vi "TxData_Organization_EVM_Max.vi"() -> ()   [LabVIEW 2023, in "ParsingData.lvlib"]
uses:
  <vilib>/Utility/file.llb/Read Delimited Spreadsheet (string).vi
  <vilib>/Utility/file.llb/Read Delimited Spreadsheet (DBL).vi
  ParsingData.lvlib
panel:
  in  "File Path":path
  out "Max EVM : Mode       Polarity                     UD att                   BFIC COM               BFIC ele                  SG Power                EIRP                           EVM":string[](array[string])
  in  "Input power_up":dbl
  in  "Input power_low":dbl
  out "EVM to EIRP":cluster{dbl[], "all rows":dbl[]}[](graph)
  out "all rows":dbl[][](array[numeric])
  out "filenames":string[](array[string])
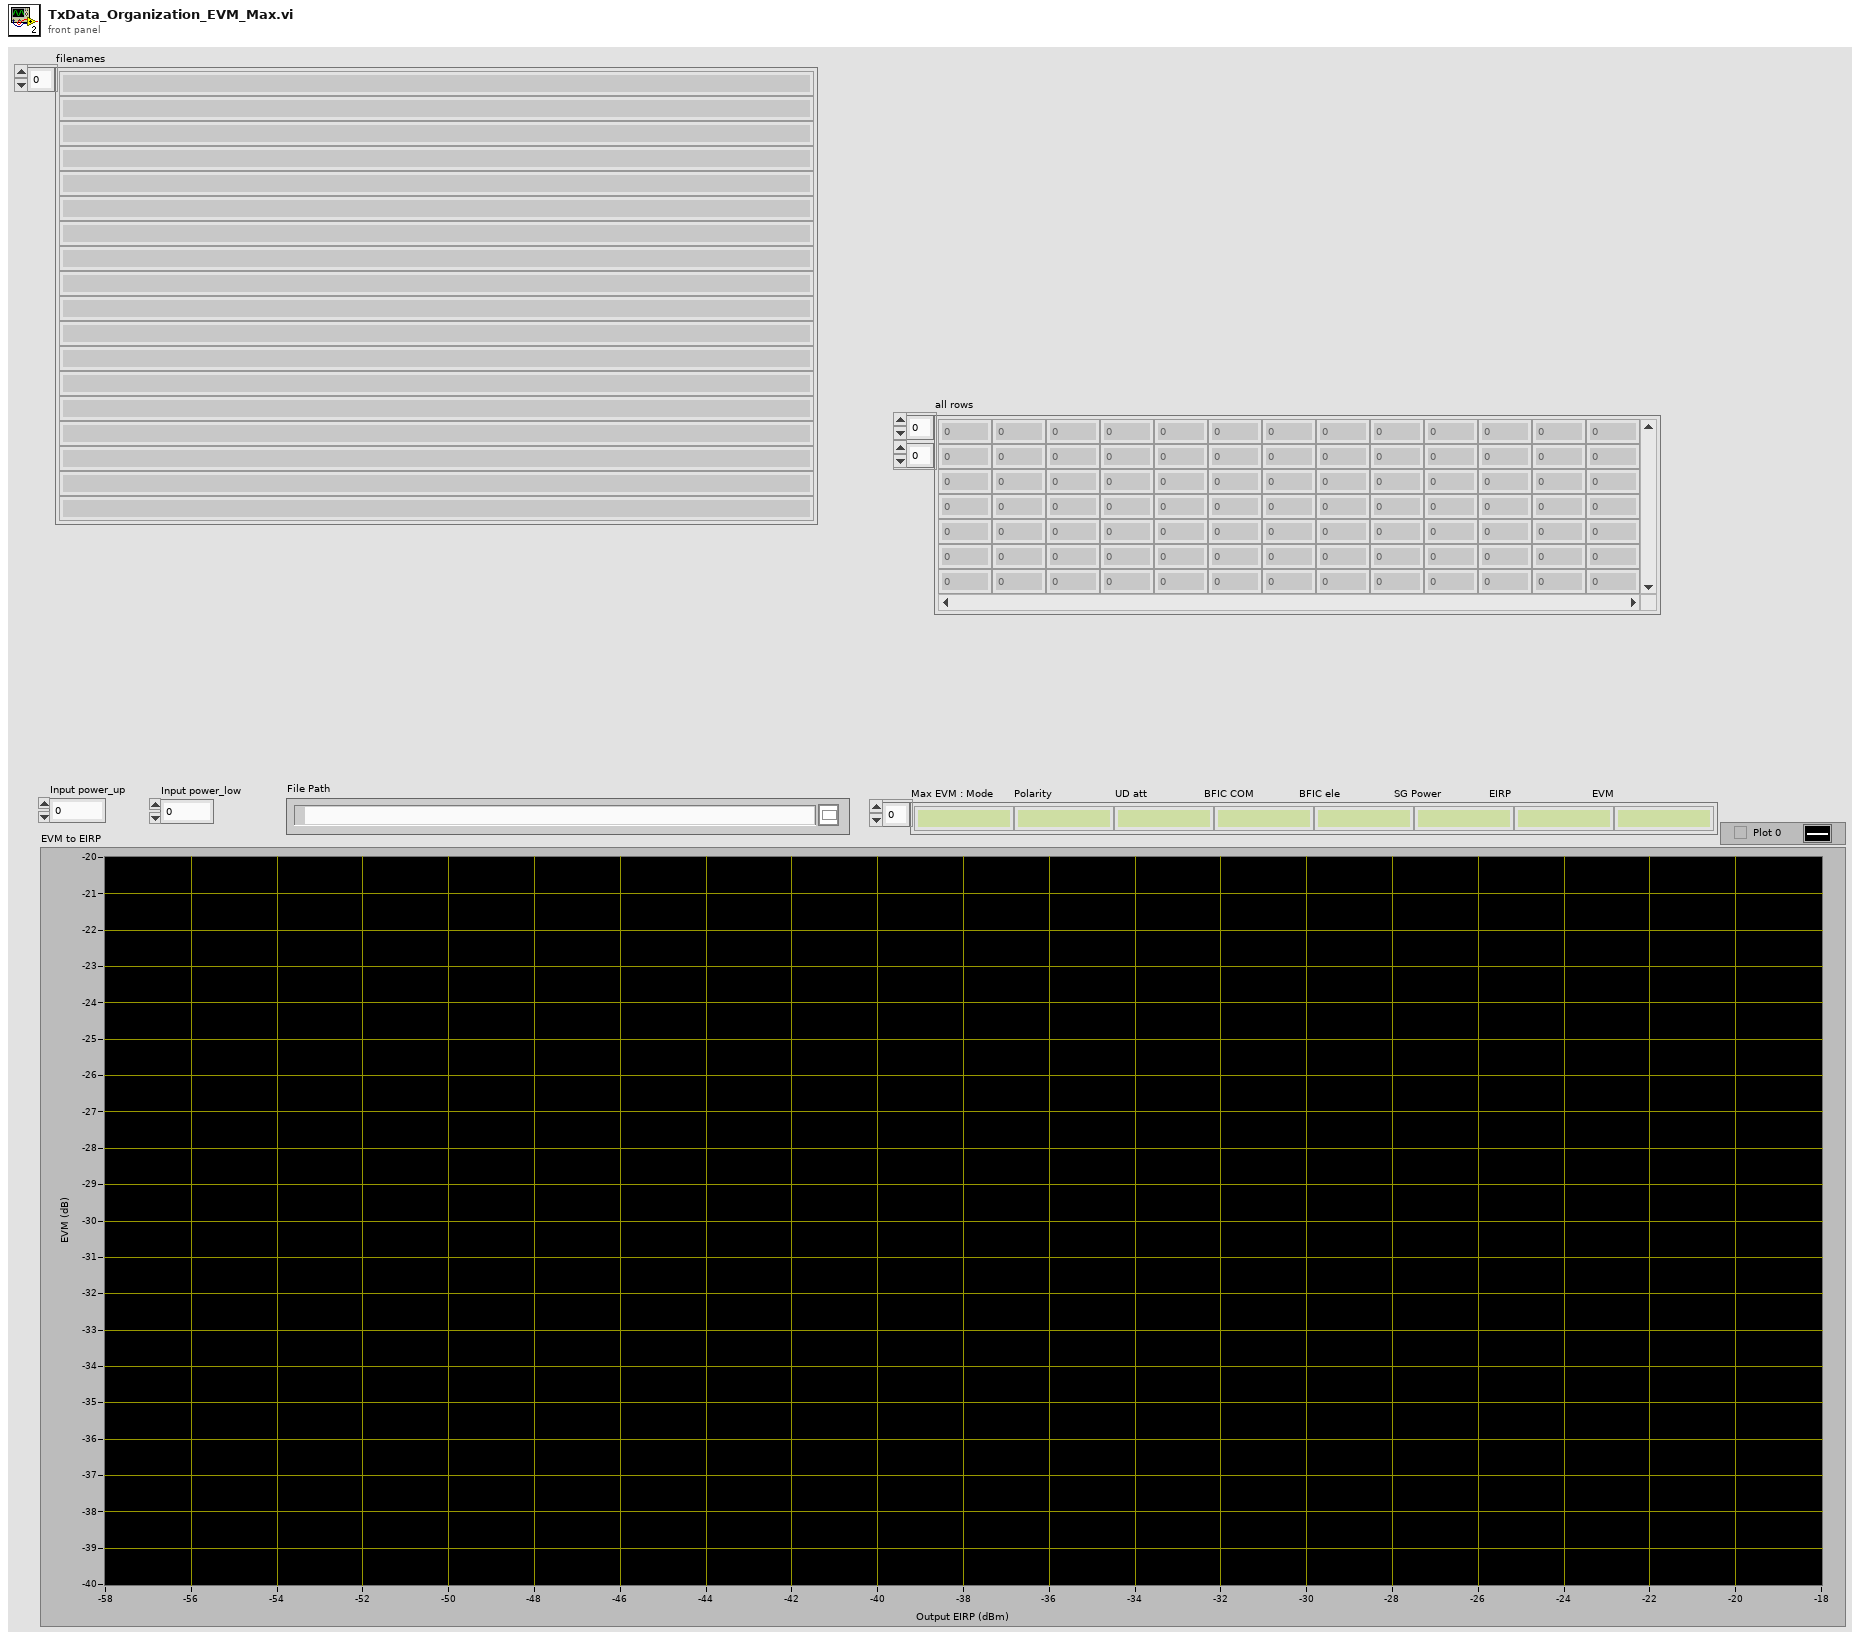
[diagram p1: front panel]
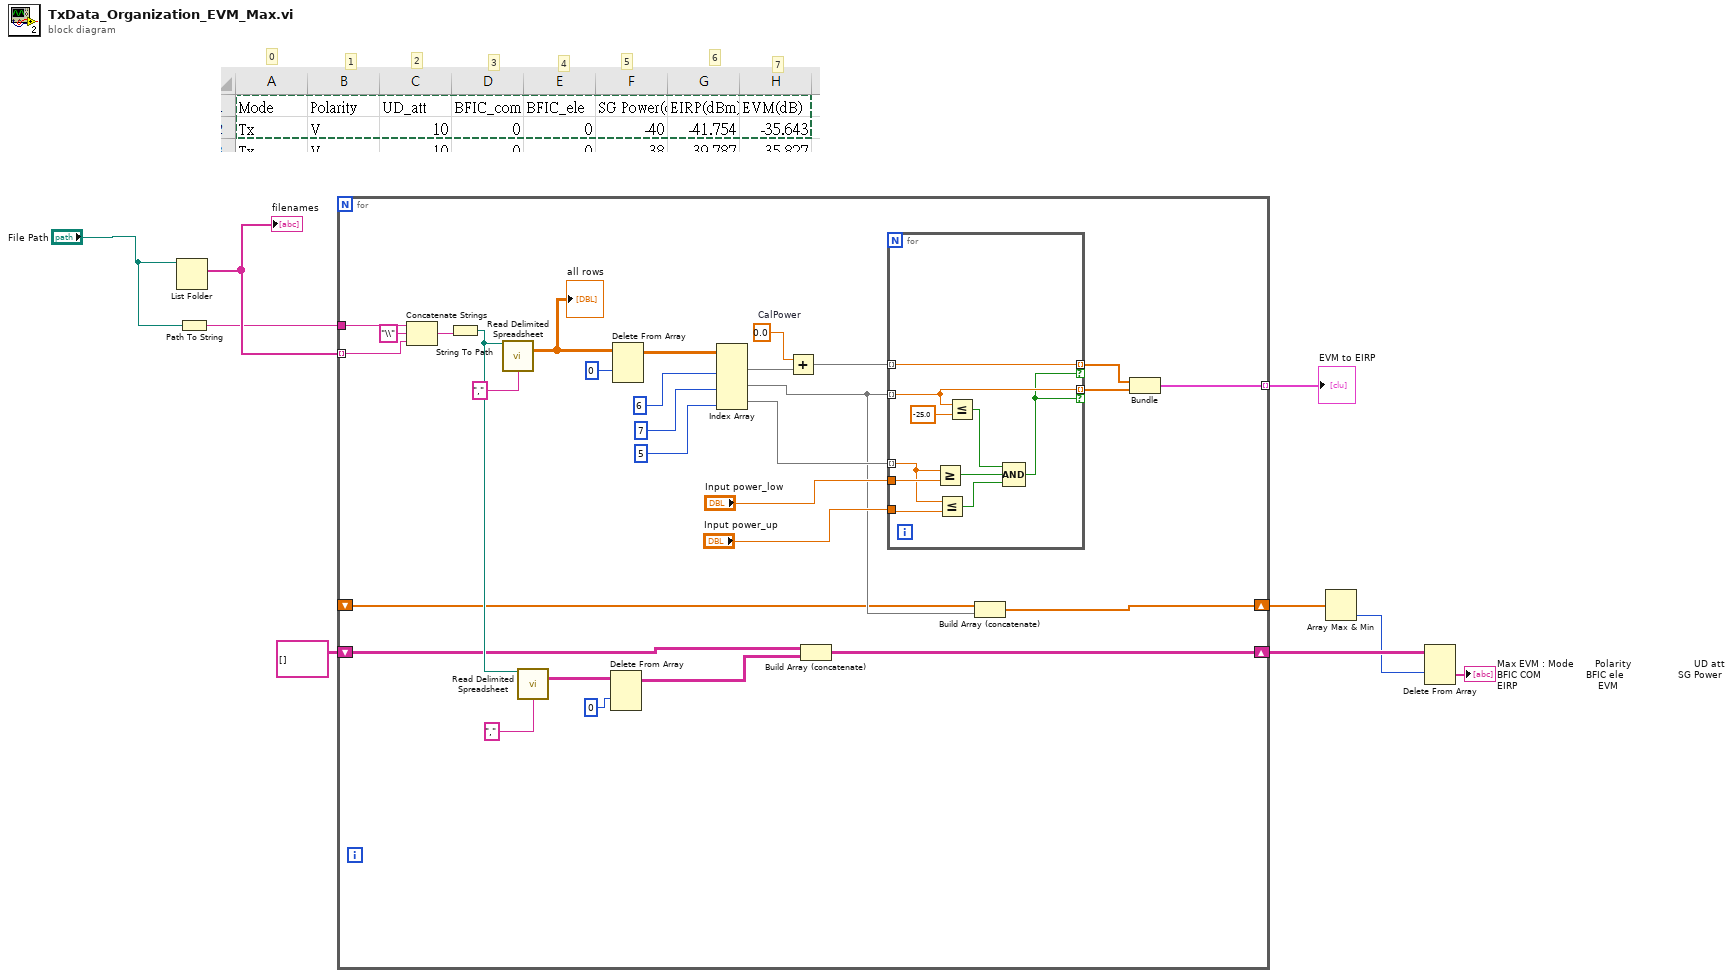
[diagram p0: block diagram]
diagram:
  # "7"
  # "6"
  # "5"
  # "4"
  # "3"
  # "2"
  # "1"
  # "0"
  n1 = List Folder(path="File Path") -> (filenames=w9:string[])  [unwired: 3 in, 3 out]
  "filenames" <- w9
  n2 = Path To String(path="File Path") -> (string=w8:string)
  n3 = for {
    tunnel: w9 -> [w36] mode=indexing
    tunnel: w8 -> [w39]
    tunnel: [w27] -> w7 mode=indexing
    shift-right: [w14] -> w4
    shift-left: string[][] [] -> [w13]
    shift-right: [w12] -> w5
    shift-left: _ -> [w10]
    w28 = 0.0  # CalPower
    n4 = Concatenate Strings(w39, "\\" ("string"), w36) -> (w38:string)
    n5 = String To Path(string=w38) -> (path=w16:path)
    n6 = call-poly <vilib>:"Read Delimited Spreadsheet.vi"("file path (dialog if empty)"=w16, "delimiter (\\t)"="," ("delimiter (\\t)")) -> ("all rows"=w34:dbl[][])  [unwired: 8 in, 5 out]
    "all rows" <- w34
    n7 = call-poly <vilib>:"Read Delimited Spreadsheet.vi"("file path (dialog if empty)"=w16, "delimiter (\\t)"="," ("delimiter (\\t)")) -> ("all rows"=w17:string[][])  [unwired: 8 in, 5 out]
    n8 = Delete From Array(array=w17, index (row)=0 ("disabled index (col)")) -> (array with subset deleted=w15:string[][])  [unwired: 2 in, 1 out]
    n9 = Delete From Array(array=w34, index (row)=0 ("disabled index (col)")) -> (array with subset deleted=w32:dbl[][])  [unwired: 2 in, 1 out]
    n10 = Index Array(array=w32, index (col) #1=6 ("disabled index (col)"), index (col) #2=7 ("index (col)"), index (col) #3=5 ("index (col)")) -> (element #1=w29:dbl[], element #2=w11:dbl[], element #3=w22:dbl[])  [unwired: 3 in]
    n11 = Add(x=w28, y=w29) -> (x+y=w26:dbl[])
    n12 = Build Array (concatenate)(w13, w15) -> (w14:string[][])
    n13 = for {
      tunnel: w26 -> [w47] mode=indexing
      tunnel: w11 -> [w48] mode=indexing
      tunnel: [w48] -> w24 mode=indexing if=w40
      tunnel: [w47] -> w25 mode=indexing if=w40
      tunnel: w22 -> [w45] mode=indexing
      tunnel: "Input power_low" -> [w46]
      tunnel: "Input power_up" -> [w44]
      n14 = Greater Or Equal?(x=w45, y=w46) -> (x >= y?=w42:bool)
      n15 = Less Or Equal?(x=w45, y=w44) -> (x <= y?=w43:bool)
      n16 = Less Or Equal?(x=w48, y=-25.0) -> (x <= y?=w41:bool)
      n17 = Compound Arithmetic op=AND(w41, w42, w43) -> (w40:bool)
    }
    n18 = Build Array (concatenate)(w10, w11) -> (w12:dbl[])
    n19 = Bundle(w25, w24) -> (w27:cluster{dbl[], dbl[]})  [unwired: 1 in]
  }
  "EVM to EIRP" <- w7
  n20 = Array Max & Min(array=w5) -> (min index (indices)=w3:i32)  [unwired: 3 out]
  n21 = Delete From Array(array=w4, index (row)=w3) -> (deleted portion=→"Max EVM : Mode       Polarity                     UD att                   BFIC COM               BFIC ele                  SG Power                EIRP                           EVM":string[])  [unwired: 2 in, 1 out]
